vi "RIGOL DG4000 Series Standard Waveform.vi"() -> ()   [LabVIEW 2015]
doc: "This example shows how to generate a standard waveform."
uses:
  <instrlib>/RIGOL DG4000 Series/Public/Configure/Configure Standard Waveform(Sine).vi
  <instrlib>/RIGOL DG4000 Series/RIGOL DG4000 Series.lvlib
panel:
  in  "DC Offset (0.00 V)":dbl
  in  "Frequency (1000 Hz)":dbl=1000.0
  in  "Amplitude (0.1 Vpp)":dbl=0.1
  in  "VISA resource name":refnum<visa-resource-name>
  # "(c) 2012 National Instruments.  ALL RIGHTS RESERVED."
  # "To change the standard waveform shape, select the corresponding poly-subVI of the Configure Standard Waveform.vi in block diagram. It is Sine by default."
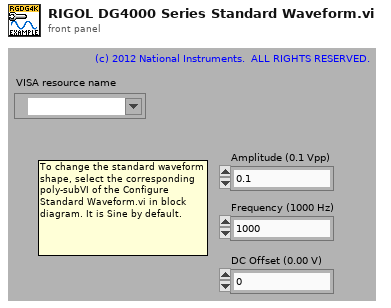
[diagram p1: front panel]
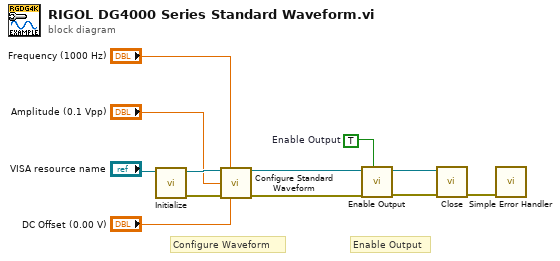
[diagram p0: block diagram]
diagram:
  w1 = TRUE  # Enable Output
  # "Enable Output"
  # "Configure Waveform"
  n1 = call "Initialize.vi"("VISA resource name"="VISA resource name") -> ("error out"=w10:errorcluster, "VISA resource name out"=w11:refnum<visa-resource-name>)  [unwired: 4 in, 5 out]
  n2 = call-poly <instrlib>:"Configure Standard Waveform.vi"("VISA resource name"=w11, "Frequency (1000 Hz)"="Frequency (1000 Hz)", "Amplitude (5 Vpp)"="Amplitude (0.1 Vpp)", "error in (no error)"=w10, "Offset (0)"="DC Offset (0.00 V)") -> ("VISA resource name out"=w6:refnum<visa-resource-name>, "error out"=w5:errorcluster)  [unwired: 3 in, 6 out]
  n3 = call "Enable Output.vi"("Enable Output (T: Enable)"=w1, "error in (no error)"=w5, "VISA resource name"=w6) -> ("error out"=w3:errorcluster, "VISA resource name out"=w4:refnum<visa-resource-name>)  [unwired: 1 in, 6 out]
  n4 = call <instrlib>:"Close.vi"("error in (no error)"=w3, "VISA resource name"=w4) -> ("error out"=w7:errorcluster)  [unwired: 9 out]
  n5 = call <vilib>:"Simple Error Handler.vi"("error in (no error)"=w7) -> ()  [unwired: 1 in, 8 out]
